vi "EnumerateAllPages.vi"(8 "error in (no error)":errorcluster, 11 "Pages":refnum<vi>[](array[refnum])) -> (0 "error out":errorcluster, 1 "#ofSubPages":i32[](array[numeric]), 2 "#ofMainPages":i32, 4 "SubPageLabels":string[](array[string]), 5 "MainPageLabels":string[](array[string]))   [LabVIEW 2013, in "RHA.lvlib"]
doc: "Enumerates both Main and Inner pages, and provides the labels for each."
uses:
  <userlib>/_OpenG.lib/array/array.llb/Filter 1D Array with Scalar (String)__ogtk.vi
  RHA.lvlib
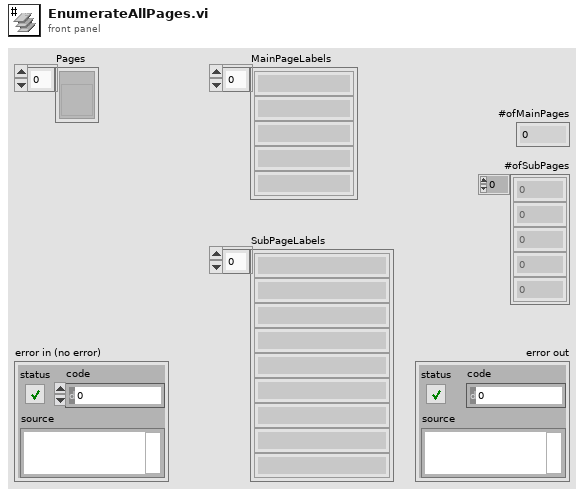
[diagram p1: front panel]
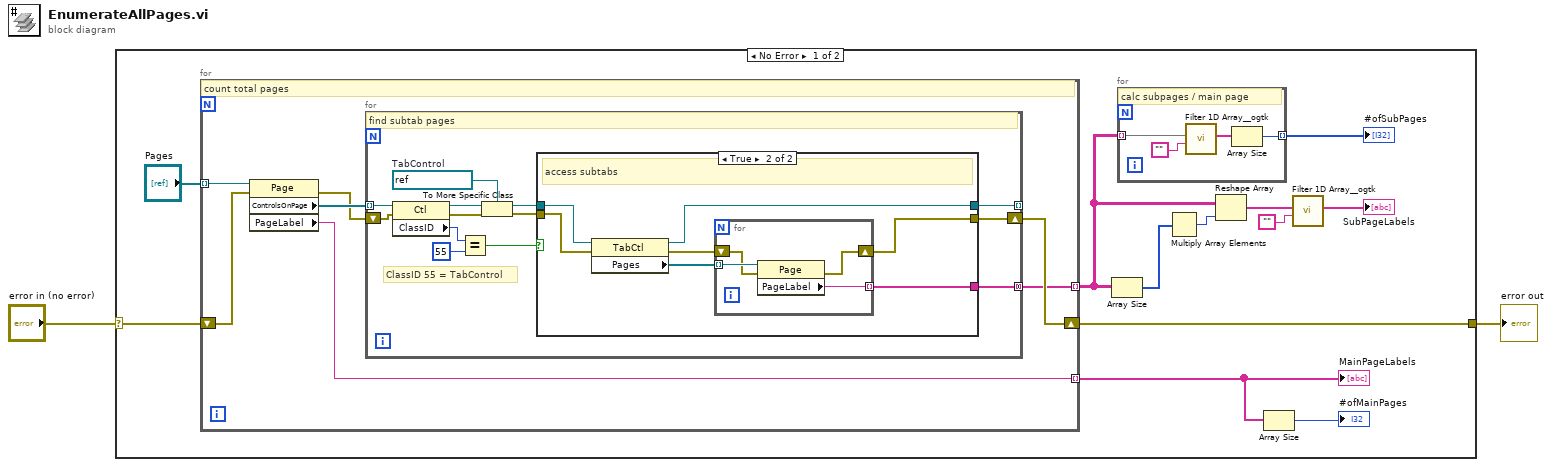
[diagram p0: block diagram]
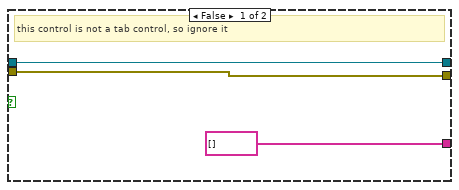
[diagram p2: hidden frame]
diagram:
  n1 = case shown="No Error" "error in (no error)" {
    selector: "error in (no error)" -> [w10 w53]
    tunnel: [w11 w53] -> w1
    frame No Error {
      n2 = for {
        tunnel: "Pages" -> [w22] mode=indexing
        tunnel: [w24] -> w13 mode=indexing
        shift-right: [w20] -> w11
        shift-left: w10 -> [w21]
        tunnel: [w19] -> w4 mode=indexing
        # "count total pages"
        n3 = property class="Page"(reference=w22, error in=w21) -> (error out=w23:errorcluster, "ControlsOnPage"=w25:refnum<vi>[], "PageLabel"=w24:string)  [unwired: 1 out]
        n4 = for {
          tunnel: w25 -> [w38] mode=indexing
          shift-right: [w32] -> w20
          shift-left: w23 -> [w35]
          tunnel: [w33] -> _ mode=indexing
          tunnel: [w26] -> w19 mode=concatenating
          w27 = refnum<vi> refnum  # TabControl
          # "ClassID 55 = TabControl"
          # "find subtab pages"
          n5 = property class="Ctl"(reference=w38, error in=w35) -> (reference out=w31:refnum<vi>, error out=w29:errorcluster, "ClassID"=w37:u32)
          n6 = Equal?(x=w37, y=u32 55) -> (x = y?=w34:bool)
          n7 = To More Specific Class(target class=w27, reference=w31, error in=w29) -> (specific class reference=w30:refnum<vi>, error out=w28:errorcluster)
          n8 = case shown="True" w34 {
            tunnel: [w41 w48] -> w33
            tunnel: w30 -> [w41 w47]
            tunnel: w28 -> [w40 w46]
            tunnel: [w40 w42] -> w32
            tunnel: [string[] [] w45] -> w26
            frame False {
              # "this control is not a tab control, so ignore it"
            }
            frame True {
              # "access subtabs"
              n9 = property on="Property Node" class="TabCtl"(reference=w47, error in=w46) -> (reference out=w48:refnum<vi>, error out=w43:errorcluster, "Pages"=w44:refnum<vi>[])
              n10 = for {
                tunnel: w44 -> [w52] mode=indexing
                tunnel: [w51] -> w45 mode=indexing
                shift-right: [w49] -> w42
                shift-left: w43 -> [w50]
                n11 = property class="Page"(reference=w52, error in=w50) -> (error out=w49:errorcluster, "PageLabel"=w51:string)  [unwired: 1 out]
              }
            }
          }
        }
      }
      "MainPageLabels" <- w13
      n12 = Array Size(array=w4) -> (size(s)=w9:i32[])
      n13 = for {
        tunnel: w4 -> [w17] mode=indexing
        tunnel: [w18] -> w3 mode=indexing
        # "calc subpages / main page"
        n14 = call-poly <userlib>:"Filter 1D Array__ogtk.vi"("items to filter"="" ("String"), "array"=w17) -> ("filtered array"=w15:string[])  [unwired: 4 in, 1 out]
        n15 = Array Size(array=w15) -> (size(s)=w18:i32)
      }
      "#ofSubPages" <- w3
      n16 = Multiply Array Elements(1:w9) -> (0:w8:i32)
      n17 = Reshape Array(w4, w8) -> (w7:string[])
      n18 = Array Size(array=w13) -> (size(s)=→"#ofMainPages":i32)
      n19 = call-poly <userlib>:"Filter 1D Array__ogtk.vi"("items to filter"="" ("String"), "array"=w7) -> ("filtered array"=→"SubPageLabels":string[])  [unwired: 4 in, 1 out]
    }
    frame Error {
    }
  }
  "error out" <- w1
